vi "Run VI Golden DUT.vi"(0 "error out":errorcluster) -> (2 "Result":string)   [LabVIEW 2014]
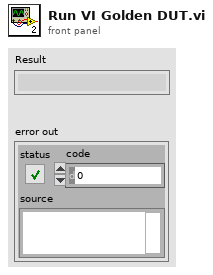
[diagram p1: front panel]
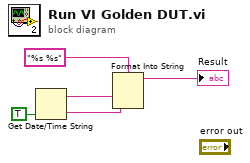
[diagram p0: block diagram]
diagram:
  n1 = Get Date/Time String(want seconds? (F)=TRUE) -> (date string=w3:string, time string=w2:string)  [unwired: 2 in]
  n2 = Format Into String(format string="%s %s", w3, w2) -> (resulting string=→"Result":string)  [unwired: 2 in, 1 out]
